vi "TCL Select Base Fragments 1frag1criterium.vi"(3 "error in (no error)":errorcluster, 4 "criterium":T1={"fragment"="", "values"=[], "operator"="is equal to"}, 5 "fragment":string) -> (0 "error out":errorcluster, 1 "matches":string[][](array[string]), 2 "fragments out":string[](array[string]))   [LabVIEW 2010]
uses:
  TCL Global.vi
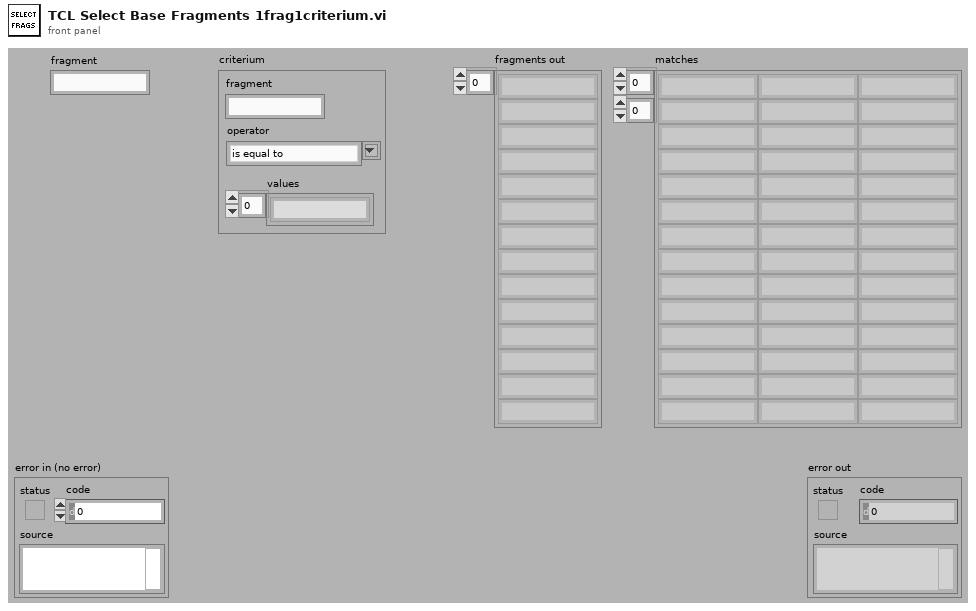
[diagram p1: front panel]
types:
  T1 = cluster{"fragment":string, "values":string[], "operator":string}
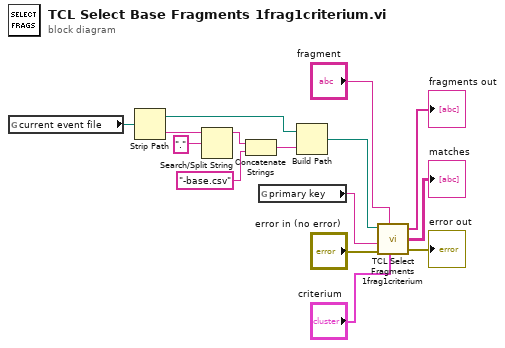
[diagram p0: block diagram]
diagram:
  n1 = global read "TCL Global.vi" "current event file"() -> (w8:path)
  n2 = Strip Path(path=w8) -> (stripped path=w7:path, name=w6:string)
  n3 = Search/Split String(string=w6, search string/char (-)=".") -> (substring before match=w1:string)  [unwired: 1 in, 2 out]
  n4 = Concatenate Strings(w1, "-base.csv" ("string")) -> (w4:string)
  n5 = global read "TCL Global.vi" "primary key"() -> (w9:string)
  n6 = Build Path(base path=w7, name or relative path=w4) -> (appended path=w3:path)
  n7 = call "TCL Select Fragments 1frag1criterium.vi"("event file"=w3, "fragment"="fragment", "primary key"=w9, "criterium"="criterium", "error in (no error)"="error in (no error)") -> ("fragments out"=→"fragments out":string[], "matches"=→"matches":string[][], "error out"=→"error out":errorcluster)  [unwired: 1 in]
